vi "Replace LastResp Token.vi"(1 "LastResp":string, 2 "Argument":string) -> (6 "Argument Out":string)   [LabVIEW 2017, in "CSM Shared.lvlib"]
uses:
  CSM Shared.lvlib
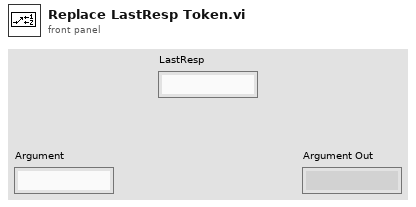
[diagram p1: front panel]
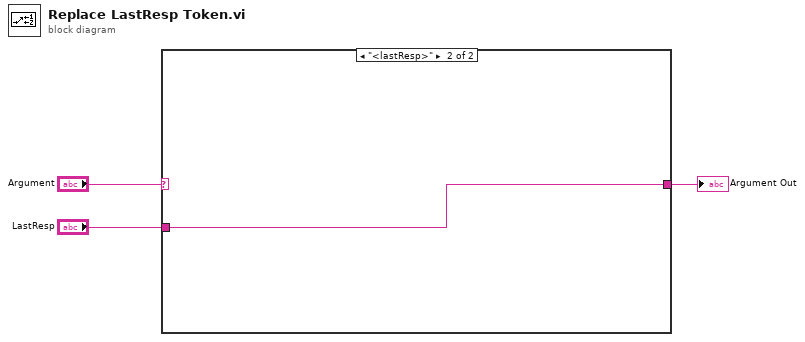
[diagram p0: block diagram]
diagram:
  n1 = case shown="\"<lastResp>\"" "Argument" {
    selector: "Argument" -> [w4 _]
    tunnel: [w4 w5] -> w2
    tunnel: "LastResp" -> [_ w5]
    frame Default {
    }
    frame "<lastResp>" {
    }
  }
  "Argument Out" <- w2
